vi "XPert IP Modem Connect.vi"() -> ()   [LabVIEW 2016]
panel:
  in  "Port":u16=23
  in  "Command":string
  in  "connection ID":refnum<k5>
  in  "error in":errorcluster
  out "error out":errorcluster
  out "Data Out":string
  in  "connect":bool
  in  "EXIT":bool
  in  "IP Address":string="166.130.11.173"
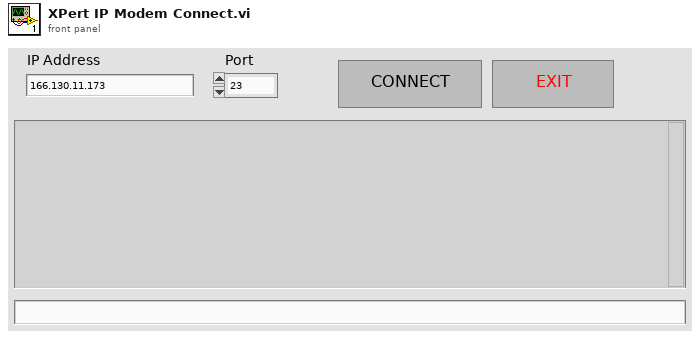
[diagram p1: front panel]
types:
  T1 = enum16{"Standard", "Buffered", "CRLF", "Immediate"}
  T2 = typedef "eventvkey.ctl" = enum16{"ASCII", "Enter", "Return", "Shift", "Ctrl", "Alt", "Cmd", "Opt", "Caps", "NumLock", "Clear", "Break", "Up", "Down", "Left", "Right", "Insert", "Delete", "Home", "End", "PageUp", "PageDown", "Escape", "Help", "Pause", "ScrollLock", "F1", "F2", "F3", "F4", "F5", "F6", "F7", "F8", "F9", "F10", "F11", "F12", "F13", "F14", "F15", "F16", "F17", "F18", "F19", "F20", "F21", "F22", "F23", "F24", "Play", "VolumeUp", "VolumeDown", "Mute", "Two Byte Char"}
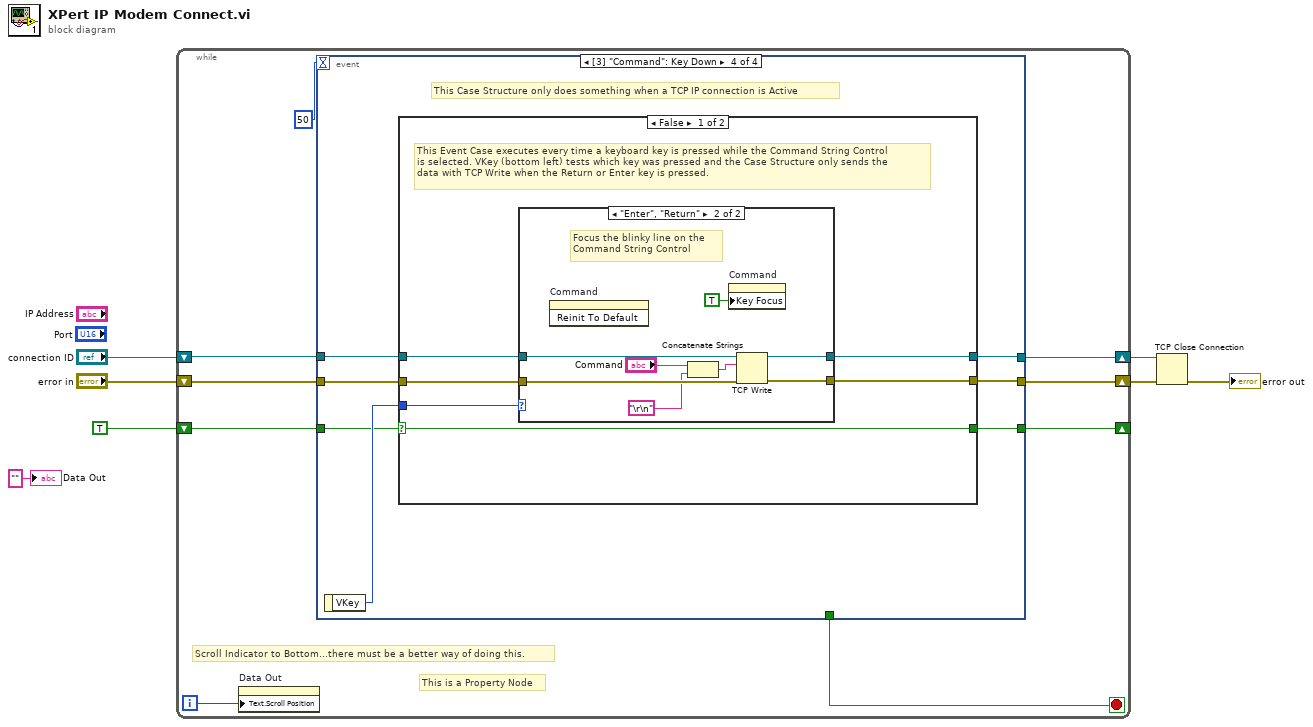
[diagram p0: block diagram]
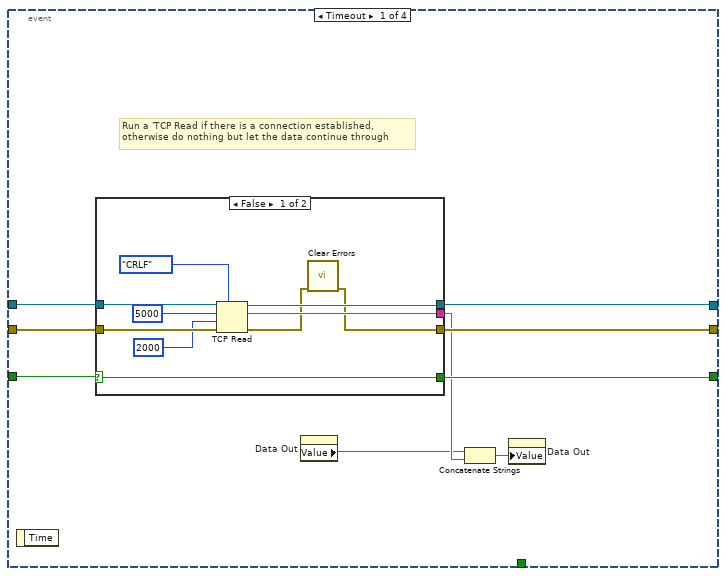
[diagram p2: hidden frame]
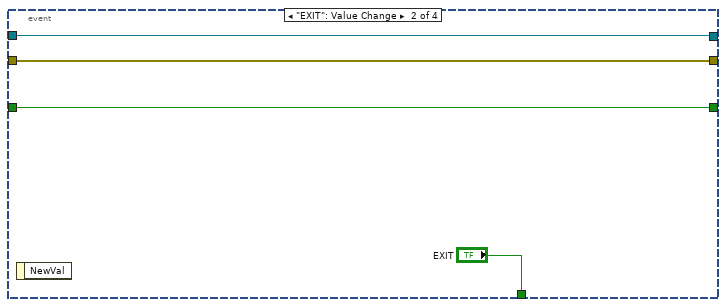
[diagram p4: hidden frame]
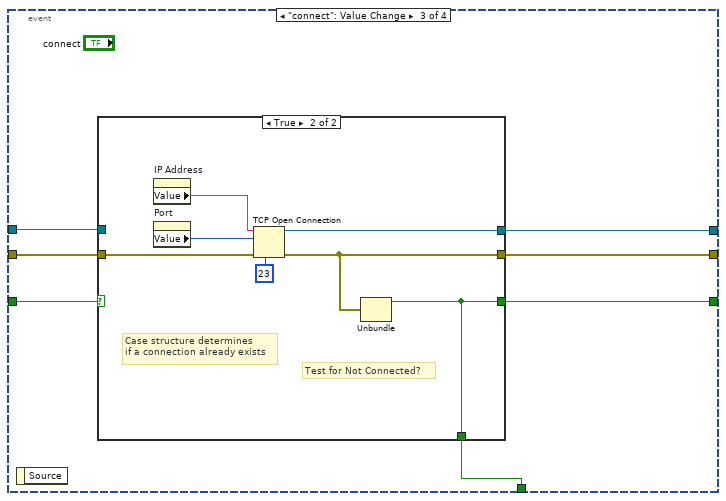
[diagram p5: hidden frame]
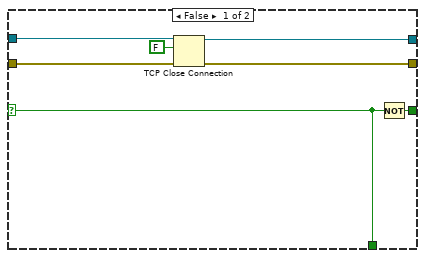
[diagram p6: hidden frame]
diagram:
  n1 = while {
    shift-right: [w13] -> w4
    shift-left: "error in" -> [w14]
    shift-right: [w12] -> w3
    shift-left: "connection ID" -> [w11]
    shift-right: [w10] -> _
    shift-left: TRUE -> [w9]
    i -> [w8]
    stop <- w16 stop-if-true
    # "This is a Property Node"
    # "Scroll Indicator to Bottom...there must be a better way of doing this."
    n2 = property on="Data Out" class="Str"("Text.Scroll Position"=w8) -> ()  [unwired: 2 in, 2 out]
    n3 = event shown="[3] \"Command\": Key Down" {
      selector: _ -> [_ _ _ _]
      dyn-events: _ -> [_ _ _ _]
      timeout: 50 -> [_ _ _ _]
      tunnel: [_ "EXIT" w43 _] -> w16
      tunnel: w14 -> [w22 w40 w49 w70]
      tunnel: [w21 w40 w47 w67] -> w13
      tunnel: [w20 w41 w48 w68] -> w12
      tunnel: w11 -> [w23 w41 w45 w69]
      tunnel: [w24 w39 w46 w64] -> w10
      tunnel: w9 -> [w25 w39 w44 w65]
      event Timeout {
        # "Run a 'TCP Read if there is a connection established, \notherwise do nothing but let the data continue through"
        n4 = event-data() -> ()  [unwired: 1 in, 1 out]
        n5 = case shown="False" w25 {
          selector: w25 -> [w35 w38]
          tunnel: [w35 w38] -> w24
          tunnel: w23 -> [w33 w36]
          tunnel: w22 -> [w34 w37]
          tunnel: [w30 _] -> w19
          tunnel: [w26 w37] -> w21
          tunnel: [w29 w36] -> w20
          frame False {
            n6 = TCP Read(connection ID=w33, bytes to read=5000, error in (no error)=w34, 7:T1."CRLF" ("mode (standard)"), 9:2000 ("timeout ms (25000)")) -> (connection ID out=w29:refnum<k5>, data out=w30:string, error out=w27:errorcluster)
            n7 = call <vilib>:"Clear Errors.vi"("error in (no error)"=w27) -> ("error out"=w26:errorcluster)  [unwired: 5 in, 1 out]
          }
          frame True {
          }
        }
        n8 = property on="Data Out" class="Str"() -> ("Value"=w18:string)  [unwired: 2 in, 2 out]
        n9 = Concatenate Strings(w18, w19) -> (w17:string)
        n10 = property on="Data Out" class="Str"("Value"=w17) -> ()  [unwired: 2 in, 2 out]
      }
      event "EXIT": Value Change {
        n11 = event-data() -> ()  [unwired: 1 in, 1 out]
      }
      event "connect": Value Change {
        n12 = event-data() -> ()  [unwired: 1 in, 1 out]
        n13 = case shown="True" w44 {
          selector: w44 -> [w50 _]
          tunnel: w49 -> [w56 w63]
          tunnel: [w53 w62] -> w48
          tunnel: [w55 w60] -> w47
          tunnel: [w51 w57] -> w46
          tunnel: w45 -> [w54 _]
          tunnel: [w50 w57] -> w43
          frame False {
            n14 = TCP Close Connection(connection ID=w54, abort (F)=FALSE, error in (no error)=w56) -> (connection ID out=w53:refnum<k5>, error out=w55:errorcluster)
            n15 = Not(x=w50) -> (.not. x?=w51:bool)
          }
          frame True {
            # "Case structure determines\nif a connection already exists"
            # "Test for Not Connected?"
            n16 = property on="IP Address" class="Str"() -> ("Value"=w59:string)  [unwired: 2 in, 2 out]
            n17 = property on="Port" class="DigNum (strict)"() -> ("Value"=w58:u16)  [unwired: 2 in, 2 out]
            n18 = TCP Open Connection(address=w59, remote port or service name=w58, local port=u16 23 ("local port (0)"), error in (no error)=w63) -> (connection ID=w62:refnum<k5>, error out=w60:errorcluster)  [unwired: 1 in]
            n19 = Unbundle(w60) -> ("status"=w57:bool)  [unwired: 2 out]
          }
        }
      }
      event "Command": Key Down {
        # "This Case Structure only does something when a TCP IP connection is Active"
        n20 = event-data() -> ("VKey"=w66:T2)  [unwired: 1 in]
        n21 = case shown="False" w65 {
          selector: w65 -> [w71 w89]
          tunnel: w70 -> [w76 w88]
          tunnel: w69 -> [w75 w87]
          tunnel: [w74 w87] -> w68
          tunnel: [w73 w88] -> w67
          tunnel: w66 -> [w72 _]
          tunnel: [w71 w89] -> w64
          frame False {
            # "This Event Case executes every time a keyboard key is pressed while the Command String Control\nis selected. VKey (bottom left) tests which key was pressed and the Case Structure only sends the \ndata with TCP Write when the Return or Enter key is pressed."
            n22 = case shown="\"Enter\", \"Return\"" w72 {
              tunnel: w76 -> [w77 w86]
              tunnel: w75 -> [w78 w85]
              tunnel: [w78 w84] -> w74
              tunnel: [w77 w83] -> w73
              frame "ASCII", Default {
              }
              frame "Enter", "Return" {
                # "Focus the blinky line on the \nCommand String Control"
                n23 = invoke on="Command" class="Str" method="Reinit To Default"() -> ()  [unwired: 3 in, 3 out]
                n24 = Concatenate Strings("Command", "\r\n") -> (w80:string)
                n25 = property on="Command" class="Str"("Key Focus"=TRUE) -> ()  [unwired: 2 in, 2 out]
                n26 = TCP Write(connection ID=w85, data in=w80, error in (no error)=w86) -> (connection ID out=w84:refnum<k5>, error out=w83:errorcluster)  [unwired: 1 in, 1 out]
              }
            }
          }
          frame True {
          }
        }
      }
    }
  }
  n27 = TCP Close Connection(connection ID=w3, error in (no error)=w4) -> (error out=→"error out":errorcluster)  [unwired: 1 in, 1 out]
  "Data Out" <- "" ("Data Out")
